vi "Search Name.vi"(9 "element":string, 11 "New Recipe.Para":T1(array[cluster])) -> (2 "x < 0?":bool, 3 "x = y?":bool)   [LabVIEW 2014, in "Master.lvclass"]
uses:
  Master/Master.lvclass
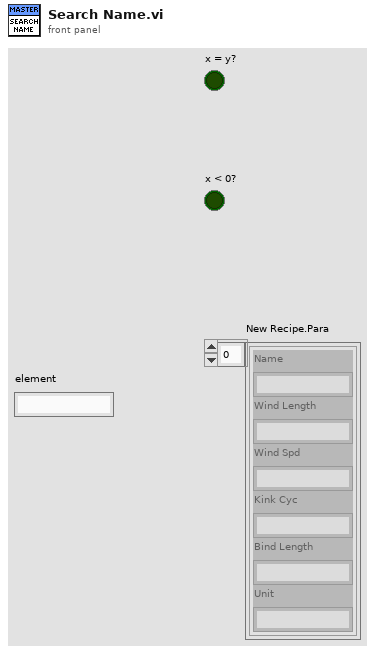
[diagram p1: front panel]
types:
  T1 = cluster{"Name":string, "Wind Length":string, "Wind Spd":string, "Kink Cyc":string, "Bind Length":string, "Unit":string}[]
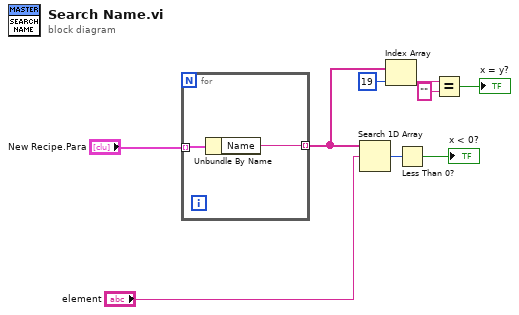
[diagram p0: block diagram]
diagram:
  n1 = for {
    tunnel: "New Recipe.Para" -> [w11] mode=indexing
    tunnel: [w10] -> w5 mode=indexing
    n2 = Unbundle By Name(w11) -> ("Name"=w10:string)
  }
  n3 = Search 1D Array(1D array=w5, element="element") -> (index of element=w8:i32)  [unwired: 1 in]
  n4 = Index Array(array=w5, index=19) -> (element=w3:string)
  n5 = Less Than 0?(x=w8) -> (x < 0?=→"x < 0?":bool)
  n6 = Equal?(x=w3, y="") -> (x = y?=→"x = y?":bool)
